vi "DataTranslation_server.vi"(0 "Board type":T1=enum."DT LV-link", 1 "interval scanning":bool, 2 "Client Time":dbl=3399992102.447224, 5 "No of samples+extra":i32=200 min=0 step=1, 7 "Trigger mode":T2, 9 "output polarity":u16(ring)=1 items=["do not change", "positive", "negative"], 11 "Ch & spans":T3[](array[typedef])=[{"high limit (10V)"=10.0, "low limit (-10V)"=-10.0, "Ch No"=0, "Var name"="RV (Vin)", "Use Latest Calib"=FALSE}] {"low limit (-10V)" format="%.3f"; "high limit (10V)" format="%.3f"}, 12 "Actual Sampling rate (Hz)":dbl=10000.0 format="%.2f", 13 "Local Client?":bool=TRUE, 14 "Current Block No":i32) -> (4 "I16 data":i16[][](array[numeric]), 6 "Block Timings":T4={"Started"=3399991568.753699, "Ended"=3399991587.0837474, "Analogue Frequency Hz"=50000.0} {"Analogue Frequency Hz" format="%.2f"}, 10 "group channel settings":T5(array[cluster])=[{"channel"="", "upper input limits"=0.0, "lower input limits"=0.0, "range"=0.0, "polarity"=0, "gain"=0.0, "coupling"=0, "input mode"=0, "scale multiplier"=1.6666666666666668e-07, "scale offset"=0.0}] {"scale offset" format="%#_16f"; "scale multiplier" format="%#_16f"; "input mode" format="%#_16f"; "coupling" format="%#_16f"; "gain" format="%#_16f"; "polarity" format="%#_16f"; "range" format="%#_16f"; "lower input limits" format="%#_16f"; "upper input limits" format="%#_16f"}, 15 "error out":errorcluster={"status"=TRUE, "code"=1172, "source"="Error calling method LvLink2.LvTask.ReadDblData2DAs1D, (System.Reflection.TargetInvocationException: Exception has been thrown by the target of an invocation.\n\tInner Exception: LvLink2.LvException: Timeout) <append><b>LvLink2.LvException</b> in OLReadMultiple2D.vi->DataTranslation_server.vi->Acquire_Data.vi->Get_data.vi->Measurement.vi"})   [LabVIEW 2010]
uses:
  Controls/Block_start_and_end.ctl
  Data_Translation/DataTranslation_global.vi
  <userlib>/LV-LINK/PolySubVIs/OLTimingSetInput.vi
  <userlib>/LV-LINK/PolySubVIs/CreateAinChan.vi
  <userlib>/LV-LINK/PolySubVIs/OLReadMultiple2D.vi
  <userlib>/LV-LINK/PolySubVIs/OLTriggerDigital.vi
  Globals/Meas_global.vi
  Controls/Ch_and_Spans.ctl
  Controls/Trigger_Mode.ctl
  Controls/Board_Types.ctl
panel:
  in  "error in":errorcluster
  out "AFG error out":errorcluster
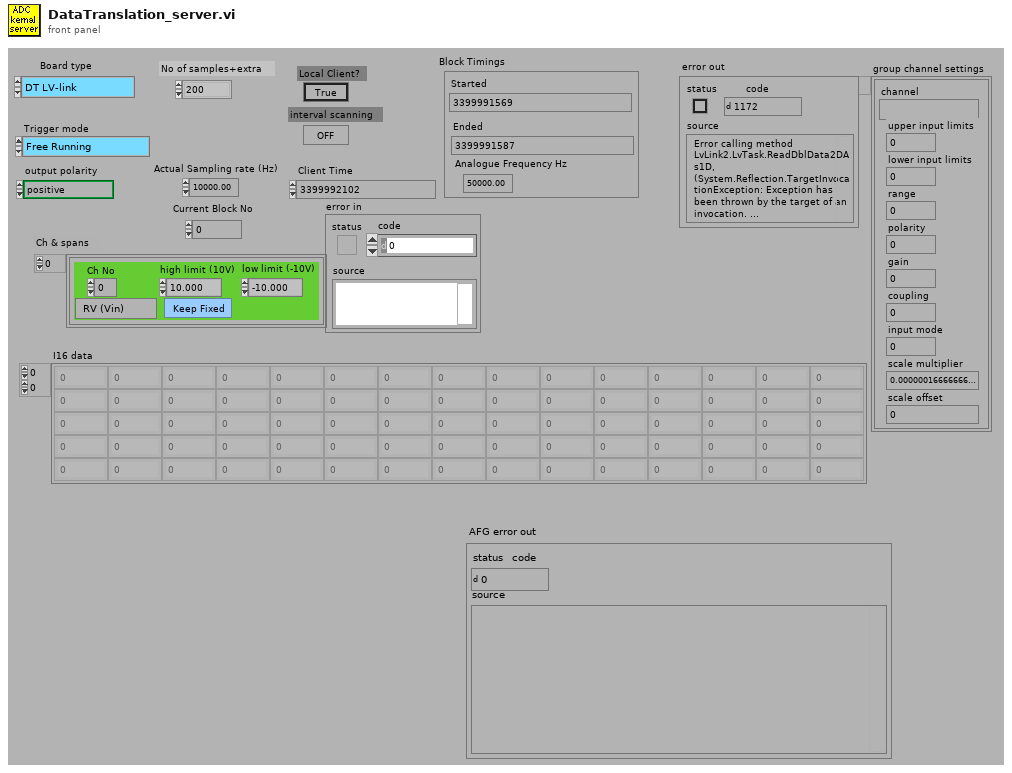
[diagram p1: front panel]
types:
  T1 = typedef "Board_Types.ctl" = enum16{"Simulate", "Local ADAM", "Server ADAM", "NI-DAQmx", "NI-DAQmxBase", "ADC488", "DT LV-link"}
  T2 = typedef "Trigger_Mode.ctl" = enum16{"Free Running", "Start on Trigger", "Trigger Every Block", "Trigger Every Sample"}
  T3 = typedef "Ch_and_Spans.ctl" = cluster{"high limit (10V)":sgl, "low limit (-10V)":sgl, "Ch No":i16, "Var name":string, "Use Latest Calib":bool}
  T4 = typedef "Block_start_and_end.ctl" = cluster{"Started":dbl, "Ended":dbl, "Analogue Frequency Hz":dbl}
  T5 = cluster{"channel":string, "upper input limits":sgl, "lower input limits":sgl, "range":sgl, "polarity":u16, "gain":sgl, "coupling":u16, "input mode":u16, "scale multiplier":dbl, "scale offset":dbl}[]
  T6 = cluster{"channel":string, "upper input limits":sgl, "lower input limits":sgl, "range":sgl, "polarity":u16, "gain":sgl, "coupling":u16, "input mode":u16, "scale multiplier":dbl, "scale offset":dbl}
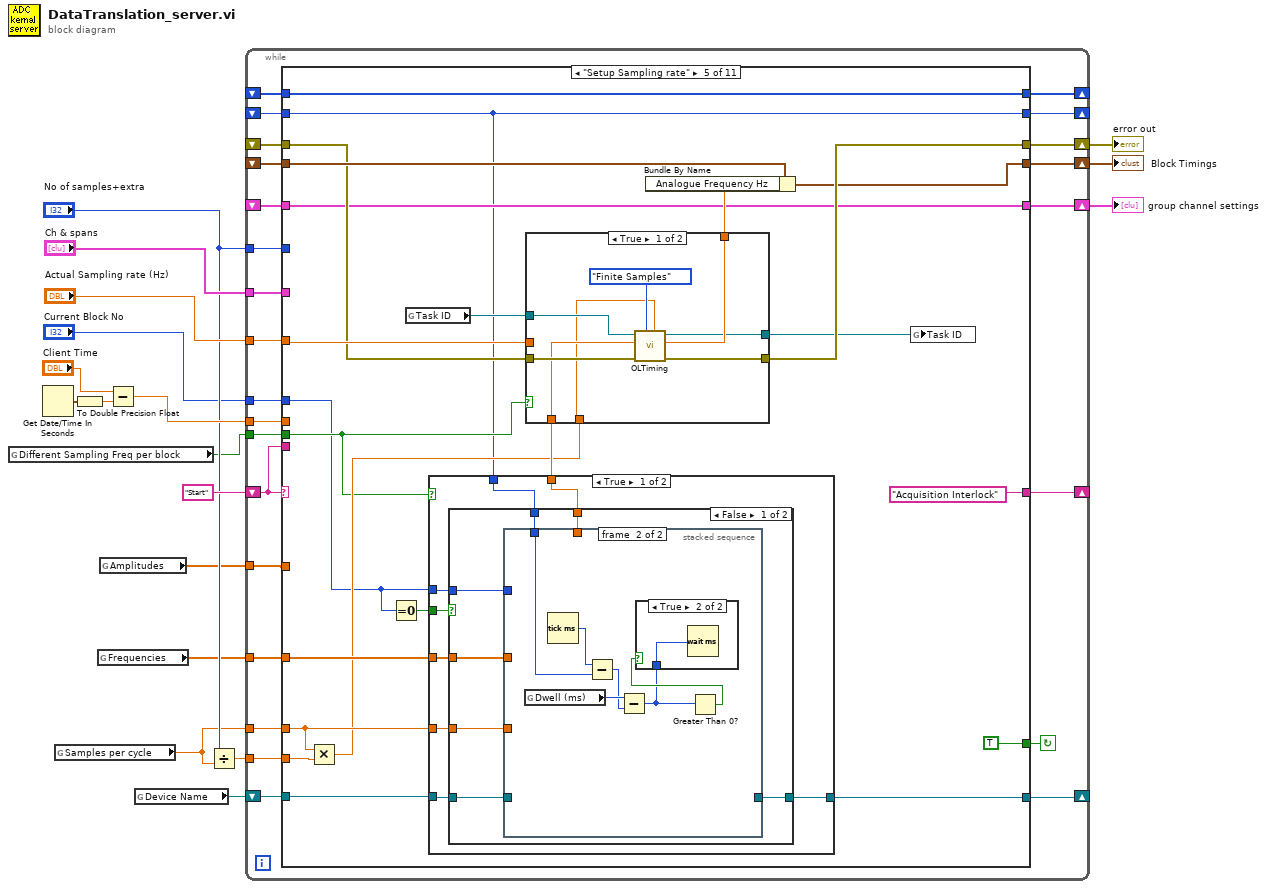
[diagram p0: block diagram]
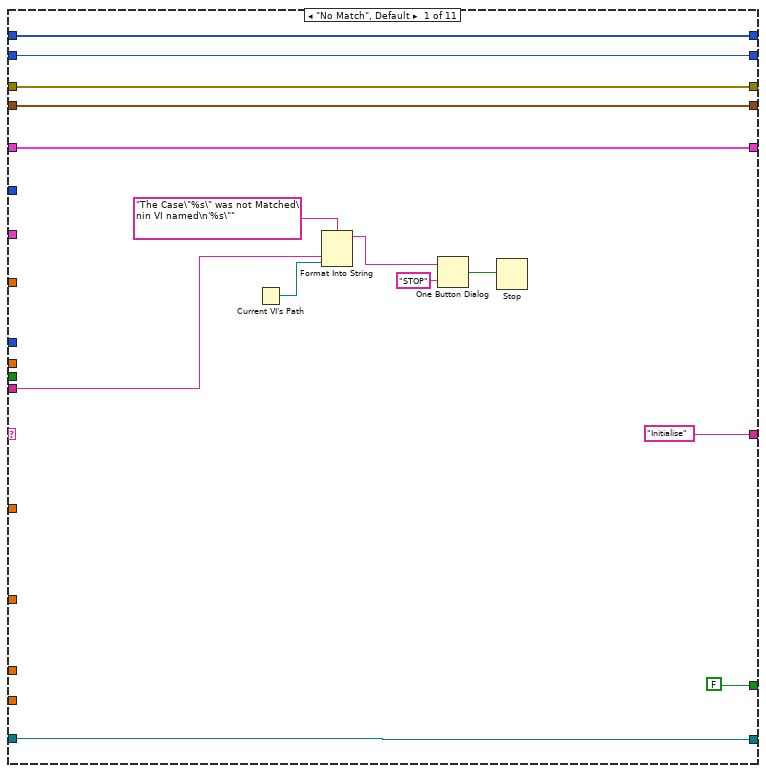
[diagram p2: hidden frame]
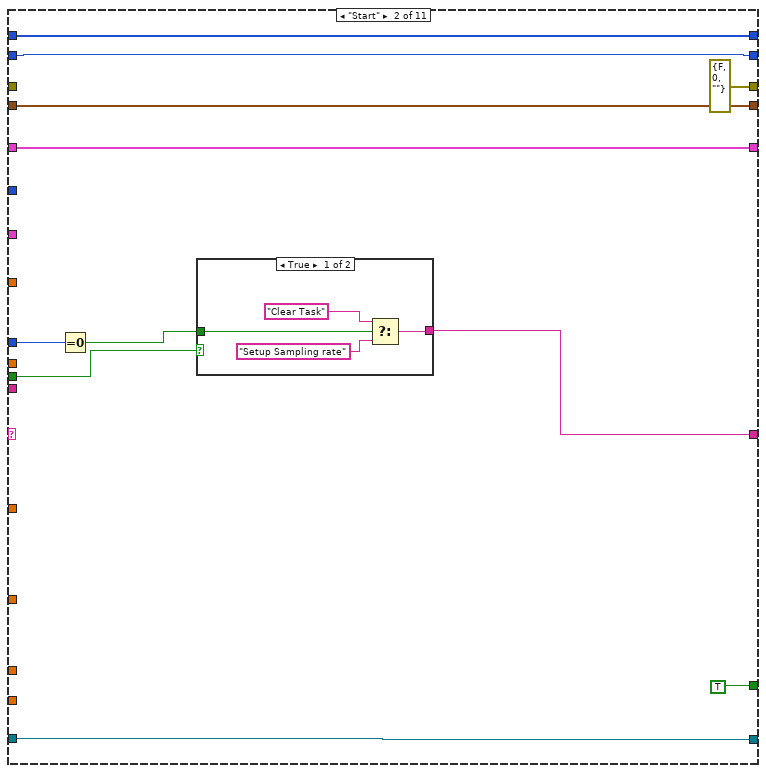
[diagram p3: hidden frame]
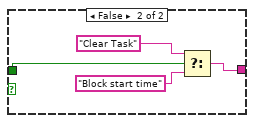
[diagram p4: hidden frame]
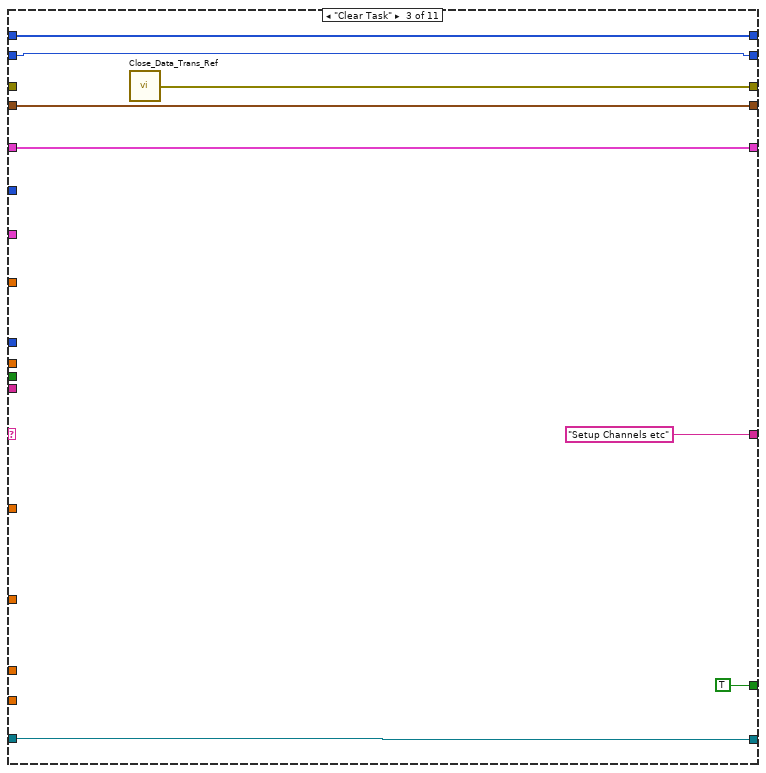
[diagram p5: hidden frame]
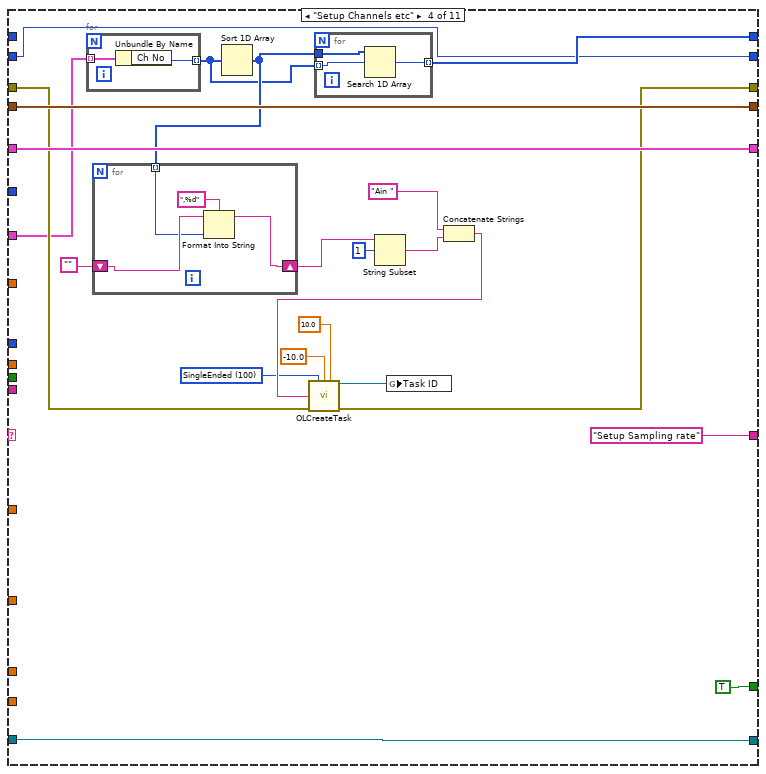
[diagram p6: hidden frame]
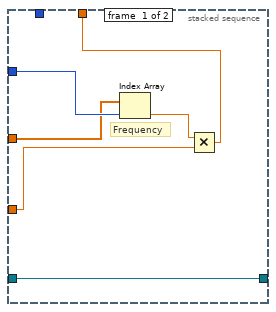
[diagram p7: hidden frame]
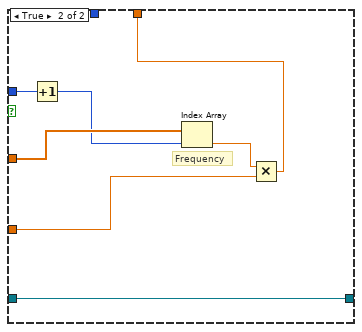
[diagram p9: hidden frame]
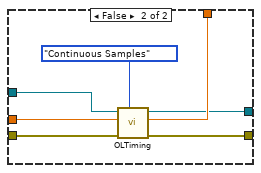
[diagram p11: hidden frame]
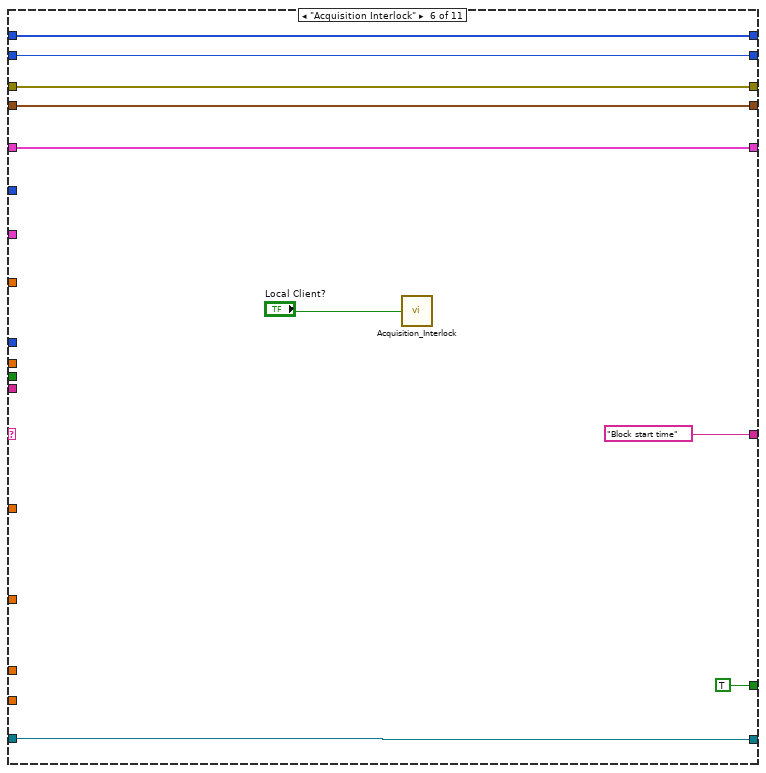
[diagram p12: hidden frame]
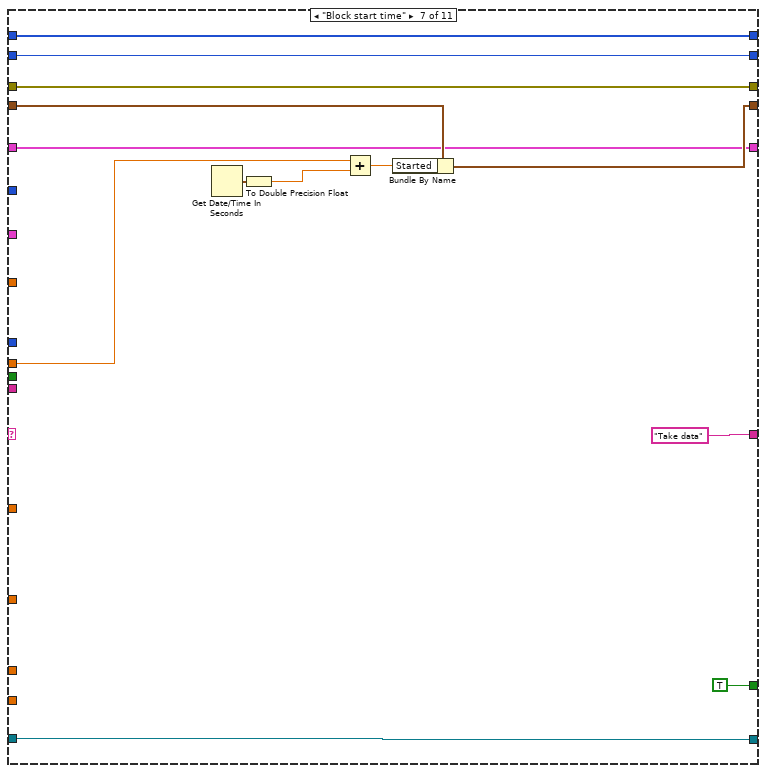
[diagram p13: hidden frame]
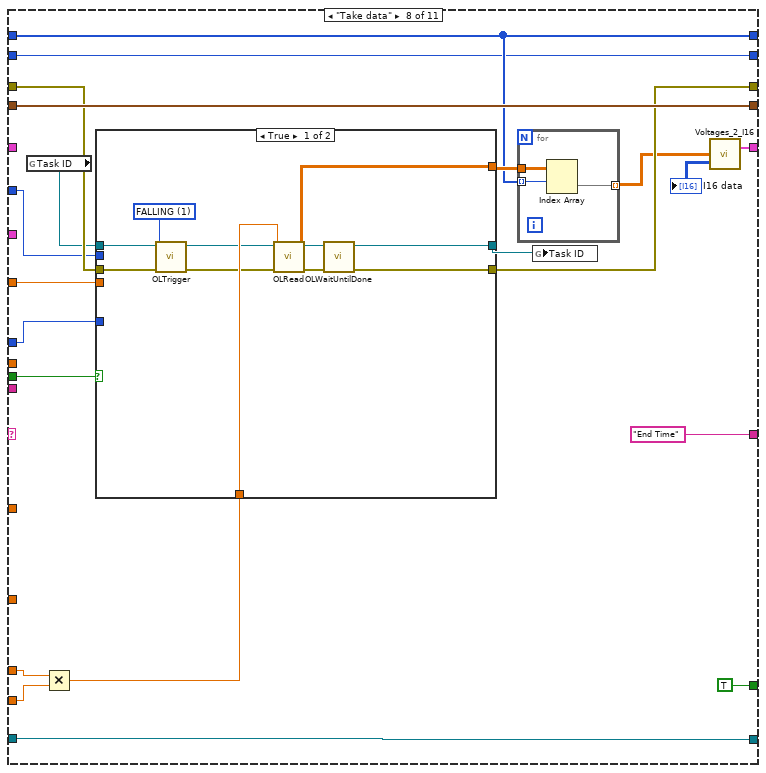
[diagram p14: hidden frame]
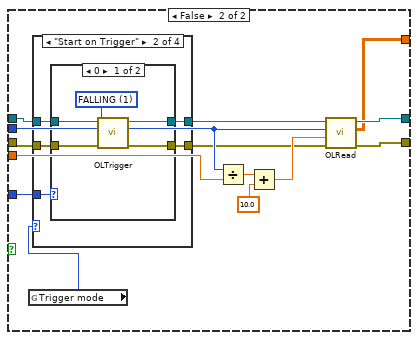
[diagram p15: hidden frame]
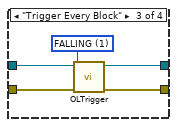
[diagram p18: hidden frame]
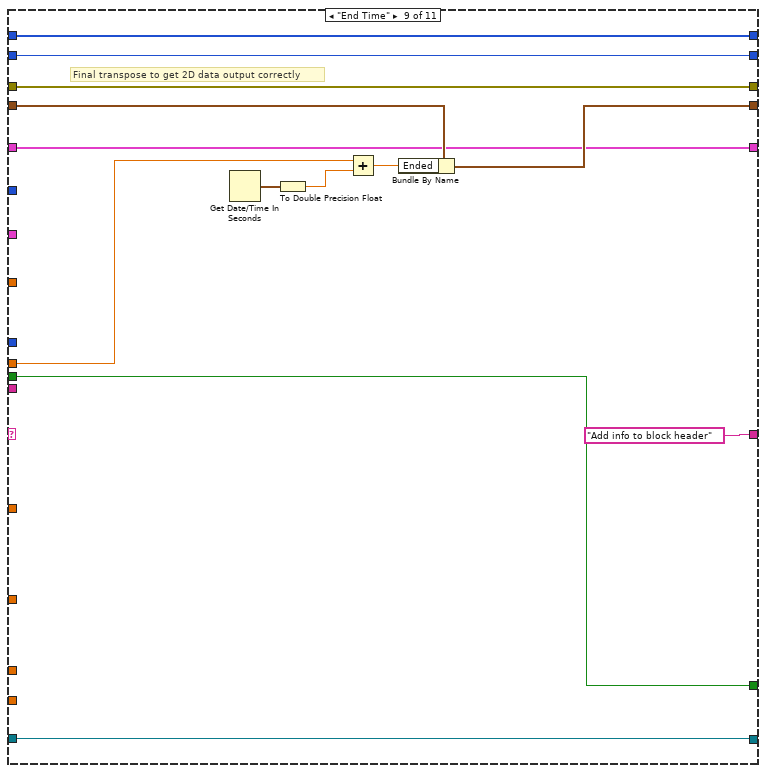
[diagram p20: hidden frame]
diagram:
  n1 = global read "DataTranslation_global.vi" "Different Sampling Freq per block"() -> (w1:bool)
  n2 = Get Date/Time In Seconds() -> (seconds since 1Jan1904=w17:timestamp)
  n3 = global read "DataTranslation_global.vi" "Samples per cycle"() -> (w4:dbl)
  n4 = To Double Precision Float(number=w17) -> (double precision float=w16:dbl)
  n5 = global read "DataTranslation_global.vi" "Frequencies"() -> (w2:dbl[])
  n6 = global read "DataTranslation_global.vi" "Amplitudes"() -> (w3:dbl[])
  n7 = Subtract(x="Client Time", y=w16) -> (x-y=w14:dbl)
  n8 = global read "DataTranslation_global.vi" "Device Name"() -> (w5:refnum<visa-resource-name>)
  n9 = Divide(x="No of samples+extra", y=w4) -> (x/y=w7:dbl)
  n10 = while {
    shift-left: "Start" -> [w41]
    shift-right: [w42] -> _
    shift-right: [w32] -> w10
    shift-left: _ -> [w40]
    shift-right: [w31] -> w11
    shift-left: _ -> [w39]
    tunnel: w14 -> [w38]
    tunnel: "Actual Sampling rate (Hz)" -> [w37]
    tunnel: "No of samples+extra" -> [w36]
    tunnel: "Current Block No" -> [w35]
    tunnel: "Ch & spans" -> [w34]
    shift-right: [w30] -> w9
    shift-left: _ -> [w33]
    shift-right: [w29] -> _
    shift-left: _ -> [w28]
    tunnel: w4 -> [w26]
    shift-right: [w25] -> _
    shift-left: w5 -> [w27]
    tunnel: w7 -> [w24]
    tunnel: w1 -> [w23]
    tunnel: w3 -> [w22]
    tunnel: w2 -> [w21]
    shift-right: [w20] -> _
    shift-left: _ -> [w19]
    stop <- w43 continue-if-true
    n11 = case shown="\"Setup Sampling rate\"" w41 {
      tunnel: [FALSE TRUE TRUE TRUE TRUE TRUE TRUE TRUE w286 FALSE FALSE] -> w43
      tunnel: ["Initialise" w64 "Setup Channels etc" "Setup Sampling rate" "Acquisition Interlock" "Block start time" "Take data" "End Time" "Add info to block header" ("f") "End" ("f") "End" ("f")] -> w42
      tunnel: w41 -> [w52 _ _ _ _ _ _ _ _ _ _]
      tunnel: [w49 errorcluster {"status"=FALSE, "code"=0, "source"=""} ("error out") w80 w87 w137 w197 w206 w227 w288 w313 w362] -> w32
      tunnel: w40 -> [w49 _ _ w94 w132 w197 w206 w228 w288 w313 w362]
      tunnel: [w47 w67 w83 w95 w134 w195 w210 w229 w293 w311 T4 {"Started"=0.0, "Ended"=0.0, "Analogue Frequency Hz"=1000.0} ("Block Timings")] -> w31
      tunnel: w39 -> [w47 w67 w83 w95 w135 w195 w211 w229 w294 w311 _]
      tunnel: w38 -> [_ _ _ _ _ _ w208 _ w285 _ _]
      tunnel: w37 -> [_ _ _ _ w136 _ _ w220 _ _ _]
      tunnel: w36 -> [_ _ _ _ _ _ _ w221 _ _ _]
      tunnel: w35 -> [_ w66 _ _ w117 _ _ w213 _ w298 _]
      tunnel: w34 -> [_ _ _ w92 _ _ _ _ _ _ _]
      tunnel: [w48 w63 w81 w104 w120 w194 w204 w230 w289 w309 w361] -> w30
      tunnel: w33 -> [w48 w63 w81 w104 w120 w194 w204 _ w289 w310 w361]
      tunnel: [w46 w61 w79 w89 w129 w193 w202 w222 w287 w312 w359] -> w29
      tunnel: w28 -> [w46 w61 w79 _ w129 w193 w202 w222 w287 w312 w359]
      tunnel: w27 -> [w45 w60 w78 w86 w126 w192 w201 w219 w284 w308 w358]
      tunnel: w22 -> [_ _ _ _ _ _ _ _ _ w303 _]
      tunnel: w21 -> [_ _ _ _ w128 _ _ _ _ w304 _]
      tunnel: w26 -> [_ _ _ _ w122 _ _ w217 _ _ _]
      tunnel: [w45 w60 w78 w86 w125 w192 w201 w219 w284 w307 w358] -> w25
      tunnel: w24 -> [_ _ _ _ w123 _ _ w218 _ _ _]
      tunnel: w23 -> [_ w59 _ _ w119 _ _ w215 w286 _ _]
      tunnel: [w44 w58 w77 w85 w118 w191 w200 w214 w283 w300 w357] -> w20
      tunnel: w19 -> [w44 w58 w77 w85 w118 w191 w200 w214 w283 _ w357]
      frame "No Match", Default {
        n12 = Current VI's Path() -> (path=w51:path)
        n13 = Format Into String(format string="The Case\"%s\" was not Matched\nin VI named\n'%s\"" ("Format String"), w52, w51) -> (resulting string=w55:string)  [unwired: 2 in, 1 out]
        n14 = One Button Dialog(message=w55, button name ("OK")="STOP") -> (true=w53:bool)
        n15 = Stop(stop? (T)=w53) -> ()
      }
      frame "Start" {
        n16 = Equal To 0?(x=w66) -> (x = 0?=w65:bool)
        n17 = case shown="True" w59 {
          tunnel: w65 -> [w70 w74]
          tunnel: [w69 w73] -> w64
          frame True {
            n18 = Select(t="Clear Task", s=w70, f="Setup Sampling rate") -> (s? t:f=w69:string)
          }
          frame False {
            n19 = Select(t="Clear Task", s=w74, f="Block start time") -> (s? t:f=w73:string)
          }
        }
      }
      frame "Clear Task" {
        n20 = call "Close_Data_Trans_Ref.vi"() -> ("Error Out"=w80:errorcluster)
      }
      frame "Setup Channels etc" {
        w93 = 100 items=["SingleEnded"=100, "Differential"=101] ("Channel Type")
        n21 = for {
          tunnel: w92 -> [w111] mode=indexing
          tunnel: [w110] -> w90 mode=indexing
          n22 = Unbundle By Name(w111) -> ("Ch No"=w110:i16)
        }
        n23 = Sort 1D Array(array=w90) -> (sorted array=w91:i16[])
        n24 = for {
          shift-right: [w113] -> w103
          shift-left: "" -> [w114]
          tunnel: w91 -> [w112] mode=indexing
          n25 = Format Into String(format string=",%d", initial string=w114, w112) -> (resulting string=w113:string)  [unwired: 1 in, 1 out]
        }
        n26 = for {
          tunnel: w91 -> [w109]
          tunnel: w90 -> [w108] mode=indexing
          tunnel: [w107] -> w89 mode=indexing
          n27 = Search 1D Array(1D array=w109, element=w108) -> (index of element=w107:i32)  [unwired: 1 in]
        }
        n28 = String Subset(string=w103, offset (0)=1) -> (substring=w100:string)  [unwired: 1 in]
        n29 = Concatenate Strings("Ain ", w100) -> (w98:string)
        n30 = call-poly <userlib>:"OLCreateTask.vi"("Channel Type"=w93, "Range Min"=-10.0, "Range Max"=10.0, "Channel"=w98, "error in (no error)"=w94) -> ("Task Out"=w88:refnum<k24>, "error out"=w87:errorcluster)  [unwired: 9 in]
        n31 = global write "DataTranslation_global.vi" "Task ID"(w88) -> ()
      }
      frame "Setup Sampling rate" {
        n32 = Multiply(x=w122, y=w123) -> (x*y=w121:dbl)
        n33 = Equal To 0?(x=w117) -> (x = 0?=w116:bool)
        n34 = global read "DataTranslation_global.vi" "Task ID"() -> (w130:refnum<k24>)
        n35 = case shown="True" w119 {
          tunnel: w128 -> [w142 _]
          tunnel: [w146 w174] -> w127
          tunnel: w122 -> [w145 w174]
          tunnel: w117 -> [w144 _]
          tunnel: w126 -> [w143 w175]
          tunnel: [w141 w175] -> w125
          tunnel: w118 -> [w140 _]
          tunnel: w116 -> [w139 _]
          frame True {
            n36 = case shown="False" w139 {
              tunnel: [w153 w170] -> w146
              tunnel: w145 -> [w152 w169]
              tunnel: w144 -> [w147 w171]
              tunnel: w143 -> [w151 w168]
              tunnel: w142 -> [w150 w172]
              tunnel: [w149 w168] -> w141
              tunnel: w140 -> [w148 _]
              frame False {
                n37 = stacked-sequence {
                  tunnel: [w159 _] -> w153
                  tunnel: w152 -> [w158 _]
                  tunnel: w147 -> [w157 _]
                  tunnel: w151 -> [w154 _]
                  tunnel: w150 -> [w156 _]
                  tunnel: [w154 _] -> w149
                  tunnel: w148 -> [_ w164]
                  frame #0 {
                    # "Frequency"
                    n38 = Index Array(array=w156, index=w157) -> (element=w155:dbl)
                    n39 = Multiply(x=w155, y=w158) -> (x*y=w159:dbl)
                  }
                  frame #1 {
                    n40 = global read "DataTranslation_global.vi" "Dwell (ms)"() -> (w163:u32)
                    n41 = Tick Count (ms)() -> (millisecond timer value=w165:u32)
                    n42 = Subtract(x=w165, y=w164) -> (x-y=w162:u32)
                    n43 = Subtract(x=w163, y=w162) -> (x-y=w160:u32)
                    n44 = Greater Than 0?(x=w160) -> (x > 0?=w161:bool)
                    n45 = case shown="True" w161 {
                      tunnel: w160 -> [_ w166]
                      frame False {
                      }
                      frame True {
                        n46 = Wait (ms)(milliseconds to wait=w166) -> ()  [unwired: 1 out]
                      }
                    }
                  }
                }
              }
              frame True {
                # "Frequency"
                n47 = Increment(x=w171) -> (x+1=w167:i32)
                n48 = Index Array(array=w172, index=w167) -> (element=w173:dbl)
                n49 = Multiply(x=w173, y=w169) -> (x*y=w170:dbl)
              }
            }
          }
          frame False {
          }
        }
        n50 = case shown="True" w119 {
          tunnel: [w183 w190] -> w137
          tunnel: w136 -> [_ w189]
          tunnel: [w182 w188] -> w133
          tunnel: w132 -> [w181 w187]
          tunnel: [w180 w186] -> w131
          tunnel: w130 -> [w179 w185]
          tunnel: w127 -> [w177 _]
          tunnel: w121 -> [w176 _]
          frame True {
            n51 = call-poly <userlib>:"OLTiming.vi"("Samples Per Channel"=w176, "Sample Mode"=enum16{"Finite Samples", "Continuous Samples"}."Finite Samples", "error in (no error)"=w181, "Sample Freq (Hz)"=w177, "Task In"=w179) -> ("error out"=w183:errorcluster, "Actual Sample Freq"=w182:dbl, "Task Out"=w180:refnum<k24>)  [unwired: 4 in]
          }
          frame False {
            n52 = call-poly <userlib>:"OLTiming.vi"("Sample Mode"=enum16{"Finite Samples", "Continuous Samples"}."Continuous Samples", "error in (no error)"=w187, "Sample Freq (Hz)"=w189, "Task In"=w185) -> ("error out"=w190:errorcluster, "Actual Sample Freq"=w188:dbl, "Task Out"=w186:refnum<k24>)  [unwired: 5 in]
          }
        }
        n53 = Bundle By Name(cluster=w135, "Analogue Frequency Hz"=w133) -> (w134:T4)
        n54 = global write "DataTranslation_global.vi" "Task ID"(w131) -> ()
      }
      frame "Acquisition Interlock" {
        n55 = call "Acquisition_Interlock.vi"("Local Control"="Local Client?") -> ()
      }
      frame "Block start time" {
        n56 = Get Date/Time In Seconds() -> (seconds since 1Jan1904=w212:timestamp)
        n57 = To Double Precision Float(number=w212) -> (double precision float=w209:dbl)
        n58 = Add(x=w208, y=w209) -> (x+y=w207:dbl)
        n59 = Bundle By Name(cluster=w211, "Started"=w207) -> (w210:T4)
      }
      frame "Take data" {
        n60 = global read "DataTranslation_global.vi" "Task ID"() -> (w225:refnum<k24>)
        n61 = Multiply(x=w217, y=w218) -> (x*y=w216:dbl)
        n62 = case shown="True" w215 {
          tunnel: w228 -> [w235 w246]
          tunnel: [w239 w258] -> w227
          tunnel: [w240 w257] -> w226
          tunnel: w225 -> [w237 w248]
          tunnel: [w244 w256] -> w224
          tunnel: w221 -> [_ w255]
          tunnel: w220 -> [_ w254]
          tunnel: w216 -> [w243 _]
          tunnel: w213 -> [_ w245]
          frame True {
            w238 = 1 items=["RISING", "FALLING"] ("External Trigger Polarity")
            n63 = call-poly <userlib>:"OLTrigger.vi"("error in (no error)"=w235, "External Trigger Polarity"=w238, "Task In"=w237) -> ("error out"=w234:errorcluster, "Task Out"=w236:refnum<k24>)  [unwired: 7 in]
            n64 = call-poly <userlib>:"OLRead.vi"("error in (no error)"=w234, "Samples Per Channel"=w243, "Task In"=w236) -> ("error out"=w241:errorcluster, "ReadData"=w244:dbl[][], "Task Out"=w242:refnum<k24>)  [unwired: 6 in]
            n65 = call <userlib>:"OLWaitUntilDone.vi"("error in"=w241, "Task In"=w242) -> ("error out"=w239:errorcluster, "Task Out"=w240:refnum<k24>)  [unwired: 8 in]
          }
          frame False {
            n66 = global read "Meas_global.vi" "Trigger mode"() -> (w250:T2)
            n67 = case shown="\"Start on Trigger\"" w250 {
              tunnel: [w260 w262 w275 w279] -> w249
              tunnel: w248 -> [w260 w264 w277 w279]
              tunnel: [w259 w261 w274 w278] -> w247
              tunnel: w246 -> [w259 w263 w276 w278]
              tunnel: w245 -> [_ w265 _ _]
              frame "Free Running" {
              }
              frame "Start on Trigger" {
                n68 = case shown="0" w265 {
                  tunnel: w264 -> [w269 w272]
                  tunnel: w263 -> [w268 w271]
                  tunnel: [w267 w272] -> w262
                  tunnel: [w266 w271] -> w261
                  frame 0 {
                    w270 = 1 items=["RISING", "FALLING"] ("External Trigger Polarity")
                    n69 = call-poly <userlib>:"OLTrigger.vi"("error in (no error)"=w268, "External Trigger Polarity"=w270, "Task In"=w269) -> ("error out"=w266:errorcluster, "Task Out"=w267:refnum<k24>)  [unwired: 7 in]
                  }
                  frame 1, Default {
                  }
                }
              }
              frame "Trigger Every Block" {
                w273 = 1 items=["RISING", "FALLING"] ("External Trigger Polarity")
                n70 = call-poly <userlib>:"OLTrigger.vi"("error in (no error)"=w276, "External Trigger Polarity"=w273, "Task In"=w277) -> ("error out"=w274:errorcluster, "Task Out"=w275:refnum<k24>)  [unwired: 7 in]
              }
              frame "Trigger Every Sample" {
              }
            }
            n71 = Divide(x=w255, y=w254) -> (x/y=w251:dbl)
            n72 = Add(x=w251, y=10.0) -> (x+y=w253:dbl)
            n73 = call-poly <userlib>:"OLRead.vi"("error in (no error)"=w247, "Timeout"=w253, "Samples Per Channel"=w255, "Task In"=w249) -> ("error out"=w258:errorcluster, "ReadData"=w256:dbl[][], "Task Out"=w257:refnum<k24>)  [unwired: 5 in]
          }
        }
        n74 = for {
          tunnel: w222 -> [w282] mode=indexing
          tunnel: w224 -> [w281]
          tunnel: [w280] -> w223 mode=indexing
          n75 = Index Array(array=w281, index (row)=w282) -> (element=w280:dbl[])  [unwired: 1 in]
        }
        n76 = global write "DataTranslation_global.vi" "Task ID"(w226) -> ()
        n77 = call "Voltages_2_I16.vi"("Voltages"=w223) -> ("Group Channel Settings"=w230:T5, "I16 data"=→"I16 data":i16[][])
      }
      frame "End Time" {
        # "Final transpose to get 2D data output correctly"
        n78 = Get Date/Time In Seconds() -> (seconds since 1Jan1904=w295:timestamp)
        n79 = To Double Precision Float(number=w295) -> (double precision float=w292:dbl)
        n80 = Add(x=w285, y=w292) -> (x+y=w291:dbl)
        n81 = Bundle By Name(cluster=w294, "Ended"=w291) -> (w293:T4)
      }
      frame "Add info to block header" {
        n82 = global read "Meas_global.vi" "Requested No of blocks"() -> (w301:i32)
        n83 = Index Array(array=w303, index=w298) -> (element=w306:dbl)
        n84 = Index Array(array=w304, index=w298) -> (element=w305:dbl)
        n85 = Decrement(x=w301) -> (x-1=w299:i32)
        n86 = for {
          tunnel: w310 -> [w344] mode=indexing
          tunnel: [w343] -> w309 mode=indexing
          tunnel: w306 -> [w342]
          tunnel: w305 -> [w341]
          i -> [w345]
          n87 = case shown="0" w345 {
            tunnel: w344 -> [w355 w356]
            tunnel: [w349 w356] -> w343
            tunnel: w342 -> [w352 _]
            tunnel: w341 -> [w351 _]
            frame 0 {
              n88 = call "Value_to_string.vi"("Value"=w352, "Label for value"="Function_Generator_Amplitude") -> ("Output string"=w348:string)  [unwired: 1 in]
              n89 = call "Value_to_string.vi"("precision"="0", "Value"=w351, "Label for value"="Function_Generator_Frequency") -> ("Output string"=w347:string)
              n90 = Concatenate Strings(w348, w347) -> (w346:string)
              n91 = Bundle By Name(cluster=w355, "channel"=w346) -> (w349:T6)
            }
            frame 1, Default {
            }
          }
        }
        n92 = Equal?(x=w298, y=w299) -> (x = y?=w302:bool)
        n93 = case shown="False" w302 {
          tunnel: w308 -> [w328 w338]
          tunnel: [w319 w336] -> w307
          tunnel: [w321 w337] -> w296
          tunnel: w304 -> [w324 w339]
          tunnel: w303 -> [w325 w340]
          tunnel: w298 -> [w323 _]
          tunnel: [w325 w340] -> _
          tunnel: [w324 w339] -> _
          tunnel: "error in" -> [w316 w334]
          frame False {
            w329 = "SOUR1" ("input 1")
            w332 = ":%s:FREQ %.;%g;"  # Frequency Command
            w333 = ":%s:VOLT %.;%g;"  # Amplitude Command
            n94 = Increment(x=w323) -> (x+1=w322:i32)
            n95 = Index Array(array=w325, index=w322) -> (element=w327:dbl)
            n96 = Index Array(array=w324, index=w322) -> (element=w326:dbl)
            n97 = Format Into String(format string=w332, w329, w326) -> (resulting string=w330:string)  [unwired: 2 in, 1 out]
            n98 = Format Into String(format string=w333, initial string=w330, w329, w327) -> (resulting string=w331:string)  [unwired: 1 in, 1 out]
            n99 = VISA Write(VISA resource name=w328, write buffer=w331, error in (no error)=w316) -> (VISA resource name out=w320:refnum<visa-resource-name>, error out=w318:errorcluster)  [unwired: 1 out]
            n100 = VISA Write(VISA resource name=w320, write buffer="OUTP1:STAT ON", error in (no error)=w318) -> (VISA resource name out=w319:refnum<visa-resource-name>, error out=w321:errorcluster)  [unwired: 1 out]
          }
          frame True {
            n101 = VISA Write(VISA resource name=w338, write buffer="OUTP1:STAT OFF", error in (no error)=w334) -> (VISA resource name out=w336:refnum<visa-resource-name>, error out=w337:errorcluster)  [unwired: 1 out]
          }
        }
        "AFG error out" <- w296
        n102 = Tick Count (ms)() -> (millisecond timer value=w300:u32)
      }
      frame "Extra case" {
      }
    }
  }
  "Block Timings" <- w11
  "error out" <- w10
  "group channel settings" <- w9
